vi "ini Ctrl_1D Str.vi"(7 "Select":enum16{"Save", "Load"}(ring), 8 "에러 입력":errorcluster caption="에러 입력(에러 없음)", 9 "값":string[](array[string]), 10 "키":string[](array[string]), 11 "섹션":string[](array[string])) -> (0 "에러 출력":errorcluster, 1 "값":string[](array[string]), 2 "경로 출력":path)   [LabVIEW 2020]
uses:
  Controls/Cmd_File path.ctl
  Controls/Cmd_File Type.ctl
  <vilib>/Utility/config.llb/Write Key (String).vi
  <vilib>/Utility/config.llb/Read Key (String).vi
  <vilib>/Utility/config.llb/NI_LVConfig.lvlib
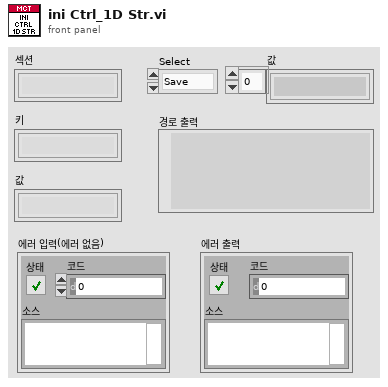
[diagram p1: front panel]
types:
  T1 = typedef "Cmd_File Type.ctl" = enum16{"엑셀", "엑셀(2003)", "텍스트", "설정", "2진", "VI", "CSV", "LOG", "폴더"}
  T2 = typedef "Cmd_File path.ctl" = enum16{"에러로그", "데이터파일경로", "성적서원본", "지난성적서", "Data Files", "경로생성", "Updater", "Template", "설정파일경로", "FTP Upload", "Update 경로", "어플리케이션"}
  T3 = typedef "NI_LVConfig.lvlib/Config Data RefNum.ctl" = refnum<k1>
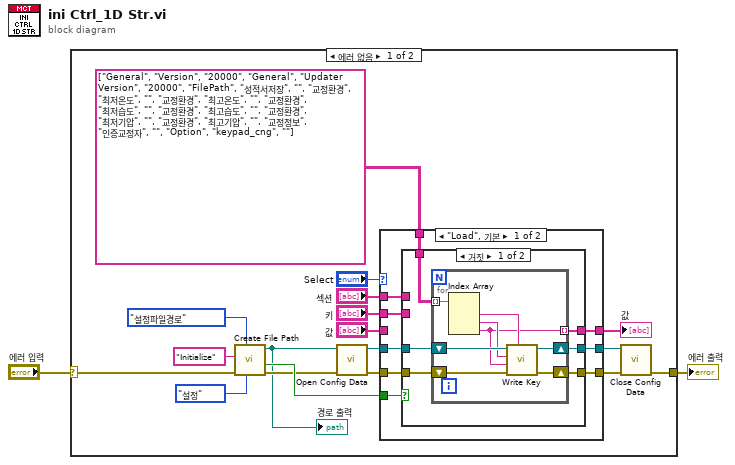
[diagram p0: block diagram]
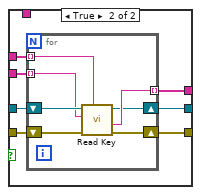
[diagram p2: hidden frame]
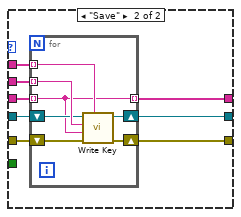
[diagram p3: hidden frame]
diagram:
  n1 = case shown="에러 없음" "에러 입력" {
    selector: "에러 입력" -> [w13 w73]
    tunnel: [w11 w73] -> w2
    frame No Error {
      n2 = call "Create File Path.vi"("파일타입"=Cmd_File_Type."설정", "항목"=Cmd_File_path."설정파일경로", "에러 입력"=w13, "문자열 in"="Initialize") -> ("error out"=w8:errorcluster, "파일존재?"=w14:bool, "파일경로"=w7:path)  [unwired: 4 in, 1 out]
      "경로 출력" <- w7
      n3 = call <vilib>:"Open Config Data.vi"("error in (no error)"=w8, "configuration file path"=w7) -> ("error out"=w5:errorcluster, "refnum"=w6:T3)  [unwired: 7 in, 1 out]
      n4 = case shown="\"Load\", 기본" "Select" {
        tunnel: [w25 w60] -> w12
        tunnel: "키" -> [w27 w65]
        tunnel: "섹션" -> [w28 w64]
        tunnel: w5 -> [w21 w63]
        tunnel: w14 -> [w29 _]
        tunnel: string[][] [["General", "Version", "20000"], ["General", "Updater Version", "20000"], ["FilePath", "성적서저장", ""], ["교정환경", "최저온도", ""], ["교정환경", "최고온도", ""], ["교정환경", "최저습도", ""], ["교정환경", "최고습도", ""], ["교정환경", "최저기압", ""], ["교정환경", "최고기압", ""], ["교정정보", "인증교정자", ""], ["Option", "keypad_cng", ""]] -> [w26 _]
        tunnel: "값" -> [_ w62]
        tunnel: [w24 w61] -> w10
        tunnel: [w23 w58] -> w9
        tunnel: w6 -> [w22 w59]
        frame "Load", Default {
          n5 = case shown="거짓" w29 {
            tunnel: w21 -> [w34 w47]
            tunnel: [w32 w45] -> w25
            tunnel: w28 -> [_ w50]
            tunnel: w27 -> [_ w49]
            tunnel: w26 -> [w35 _]
            tunnel: w22 -> [w33 w48]
            tunnel: [w31 w46] -> w24
            tunnel: [w30 w44] -> w23
            frame False {
              n6 = for {
                shift-right: [w40] -> w32
                shift-left: w34 -> [w43]
                shift-right: [w41] -> w31
                shift-left: w33 -> [w42]
                tunnel: w35 -> [w39] mode=indexing
                tunnel: [w36] -> w30 mode=indexing
                n7 = Index Array(array=w39) -> (element #1=w38:string, element #2=w37:string, element #3=w36:string)  [unwired: 3 in]
                n8 = call-poly <vilib>:"Write Key.vi"("section"=w38, "error in (no error)"=w43, "value"=w36, "key"=w37, "refnum"=w42) -> ("error out"=w40:errorcluster, "refnum out"=w41:T3)  [unwired: 4 in, 1 out]
              }
            }
            frame True {
              n9 = for {
                tunnel: w50 -> [w55] mode=indexing
                tunnel: w49 -> [w54] mode=indexing
                tunnel: [w53] -> w44 mode=indexing
                shift-right: [w51] -> w45
                shift-left: w47 -> [w57]
                shift-right: [w52] -> w46
                shift-left: w48 -> [w56]
                n10 = call-poly <vilib>:"Read Key.vi"("section"=w55, "error in (no error)"=w57, "key"=w54, "refnum"=w56) -> ("error out"=w51:errorcluster, "value"=w53:string, "refnum out"=w52:T3)  [unwired: 4 in, 1 out]
              }
            }
          }
        }
        frame "Save" {
          n11 = for {
            tunnel: w65 -> [w70] mode=indexing
            tunnel: w64 -> [w69] mode=indexing
            tunnel: w62 -> [w66] mode=indexing
            shift-right: [w72] -> w61
            shift-left: w59 -> [w68]
            shift-right: [w71] -> w60
            shift-left: w63 -> [w67]
            tunnel: [w66] -> w58 mode=indexing
            n12 = call-poly <vilib>:"Write Key.vi"("section"=w69, "error in (no error)"=w67, "value"=w66, "key"=w70, "refnum"=w68) -> ("error out"=w71:errorcluster, "refnum out"=w72:T3)  [unwired: 4 in, 1 out]
          }
        }
      }
      "값" <- w9
      n13 = call <vilib>:"Close Config Data.vi"("error in (no error)"=w12, "refnum"=w10) -> ("error out"=w11:errorcluster)  [unwired: 8 in, 1 out]
    }
    frame Error {
    }
  }
  "에러 출력" <- w2
